vi "Uart Set Baudrate.vi"(8 "error in (no error)":errorcluster, 9 "Baudrate":u32, 10 "Channel":u8, 11 "LINX Client in":refnum<class "LINX Client.lvclass">) -> (0 "error out":errorcluster, 1 "Actual Baudrate":u32, 3 "LINX Client out":refnum<class "LINX Client.lvclass">)   [LabVIEW 2020, in "LINX Client.lvclass"]
uses:
  LINX Client.lvclass
  C:/Users/rkalbermatter/Projects/LabVIEW Hobbyist/LabVIEW/vi.lib/MakerHub/LINX/API/LINX Base.lvclass
  LINX Base.lvclass
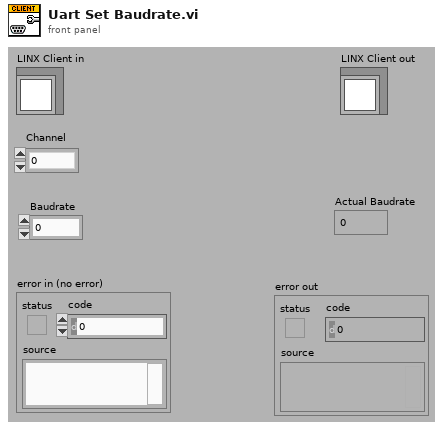
[diagram p1: front panel]
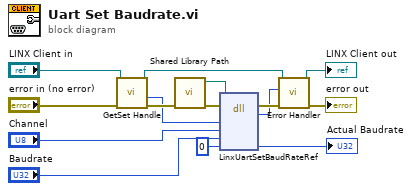
[diagram p0: block diagram]
diagram:
  n1 = call-dynamic "GetSet Handle.vi"("error in"="error in (no error)", "LINX Base in"="LINX Client in") -> ("error out"=w2:errorcluster, "handle out"=w1:u64, "LINX Base out"=w3:refnum<class "LINX Client.lvclass">)  [unwired: 3 in, 4 out]
  n2 = call "Shared Library Path.vi"("error in (no error)"=w2) -> ("error out"=w13:errorcluster, "Path"=w11:path)  [unwired: 9 out]
  n3 = dll-call lib="Z:/Development/LabVIEW Hobbyist Toolkit/LabVIEW/vi.lib/MakerHub/LINX/Resources/libLinxDevice.dll" fn="LinxUartSetBaudRateRef"(path in=w11, error in=w13, "device"=w1, "channel"="Channel", "baudrate"="Baudrate", "actualBaud"=u32 0) -> (error out=w12:errorcluster, "status"=w9:i32, "actualBaud"=→"Actual Baudrate":u32)  [unwired: 4 in, 1 out]
  n4 = call "Error Handler.vi"("error in (no error)"=w12, "LINX error code"=w9, "LINX Base in"=w3) -> ("error out"=→"error out":errorcluster, "LINX Base out"=→"LINX Client out":refnum<class "LINX Client.lvclass">)  [unwired: 1 in, 6 out]
